vi "25.Evd.10_AskEfarmog.vi"() -> ()   [LabVIEW 2020]
uses:
  <vilib>/Utility/file.llb/Write Delimited Spreadsheet (DBL).vi
panel:
  in  "file path (dialog if empty)":path
  out "current time":timestamp
  out "transposed array":dbl[][](array[numeric])
  out "Waveform Chart":dbl(graph)
  out "String":string
  in  "B":dbl
  in  "A":dbl
  in  "stop graph":bool
  out "XY Graph":cluster{dbl[], dbl[]}(graph)
  in  "main stop":bool
  out "Main Stop Pressed":bool
  in  "led stop":bool
  in  "Led On/Off (ms)":dbl
  out "Elapsed Time (ms)":dbl
  out "Elapsed Time (s)":i64
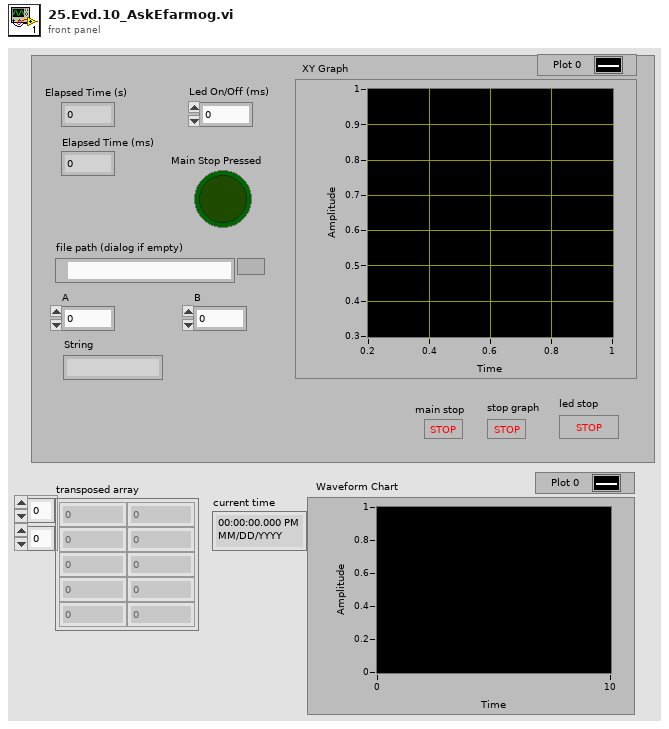
[diagram p1: front panel]
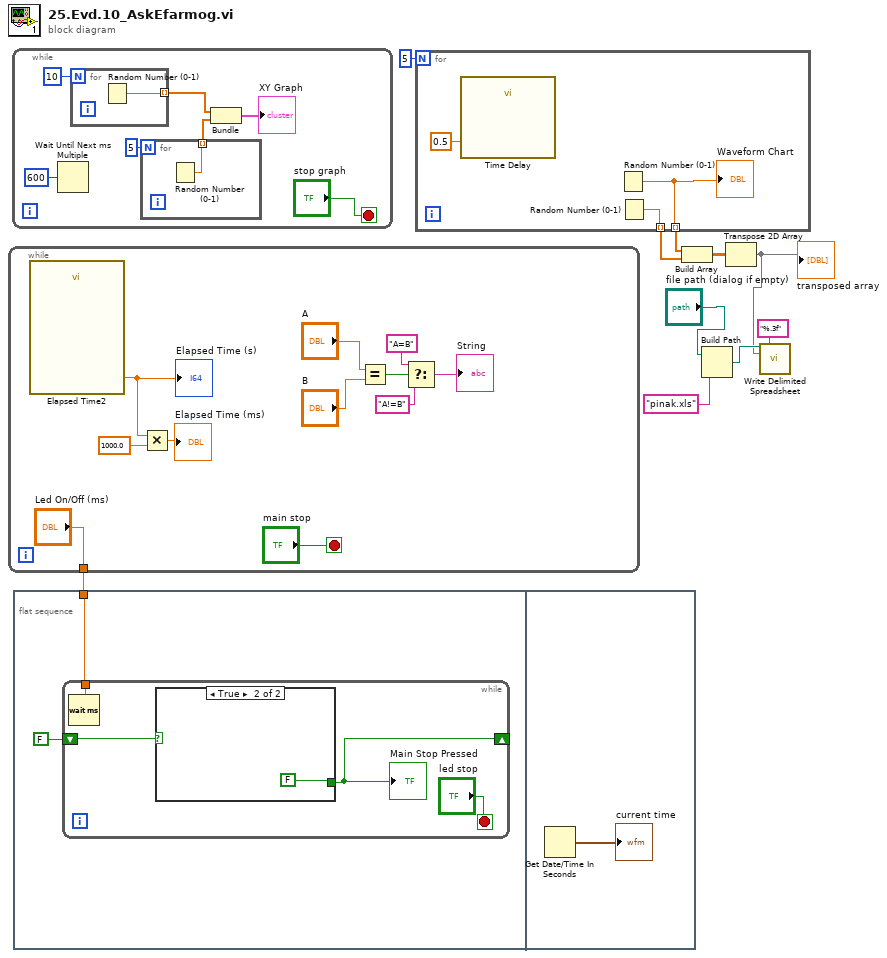
[diagram p0: block diagram]
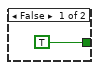
[diagram p2: hidden frame]
diagram:
  n1 = while {
    tunnel: ["Led On/Off (ms)"] -> w6
    stop <- "main stop" stop-if-true
    n2 = call "Elapsed Time2"() -> ("Elapsed Time (s)"=w21:dbl)  [unwired: 12 in, 7 out]
    "Elapsed Time (s)" <- w21
    n3 = Multiply(x=w21, y=1000.0) -> (x*y=→"Elapsed Time (ms)":dbl)
    n4 = Equal?(x="A", y="B") -> (x = y?=w14:bool)
    n5 = Select(t="A=B", s=w14, f="A!=B") -> (s? t:f=→"String":string)
  }
  n6 = while {
    stop <- "stop graph" stop-if-true
    n7 = Wait Until Next ms Multiple(millisecond multiple=u32 600) -> ()  [unwired: 1 out]
    n8 = for {
      N: 10 -> [_]
      tunnel: [w30] -> w26 mode=indexing
      n9 = Random Number (0-1)() -> (number: 0 to 1=w30:dbl)
    }
    n10 = for {
      N: 5 -> [_]
      tunnel: [w29] -> w25 mode=indexing
      n11 = Random Number (0-1)() -> (number: 0 to 1=w29:dbl)
    }
    n12 = Bundle(w26, w25) -> (→"XY Graph":cluster{dbl[], dbl[]})  [unwired: 1 in]
  }
  n13 = flat-sequence {
    tunnel: w6 -> [w31]
    frame #0 {
      n14 = while {
        shift-right: [w34] -> _
        shift-left: FALSE -> [w35]
        tunnel: w31 -> [w33]
        stop <- "led stop" stop-if-true
        n15 = Wait (ms)(milliseconds to wait=w33) -> ()  [unwired: 1 out]
        n16 = case shown="True" w35 {
          tunnel: [TRUE FALSE] -> w34
          frame False {
          }
          frame True {
          }
        }
        "Main Stop Pressed" <- w34
      }
    }
    frame #1 {
      n17 = Get Date/Time In Seconds() -> (seconds since 1Jan1904=→"current time":timestamp)
    }
  }
  n18 = for {
    N: 5 -> [_]
    tunnel: [w42] -> w9 mode=indexing
    tunnel: [w41] -> w8 mode=indexing
    n19 = call "Time Delay"("Delay Time (s)"=0.5) -> ()  [unwired: 10 in, 1 out]
    n20 = Random Number (0-1)() -> (number: 0 to 1=w42:dbl)
    "Waveform Chart" <- w42
    n21 = Random Number (0-1)() -> (number: 0 to 1=w41:dbl)
  }
  n22 = Build Array(w9, w8) -> (w7:dbl[][])
  n23 = Build Path(base path="file path (dialog if empty)", name or relative path="pinak.xls") -> (appended path=w3:path)
  n24 = Transpose 2D Array(2D array=w7) -> (transposed array=w2:dbl[][])
  "transposed array" <- w2
  n25 = call-poly <vilib>:"Write Delimited Spreadsheet.vi"("file path (dialog if empty)"=w3, "format (%.3f)"="%.3f", "2D data"=w2) -> ()  [unwired: 11 in, 2 out]
